vi "CallVI.vi"(1 "Output Names":string[](array[string]), 2 "Input Values":variant[](array[variant]), 3 "Input Names":string[](array[string]), 4 "VI":refnum<vi>) -> (0 "Output Values":variant[](array[variant]))   [LabVIEW 2014]
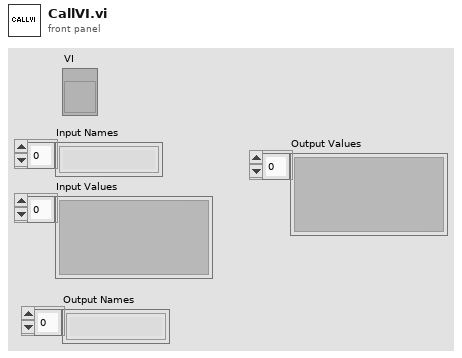
[diagram p1: front panel]
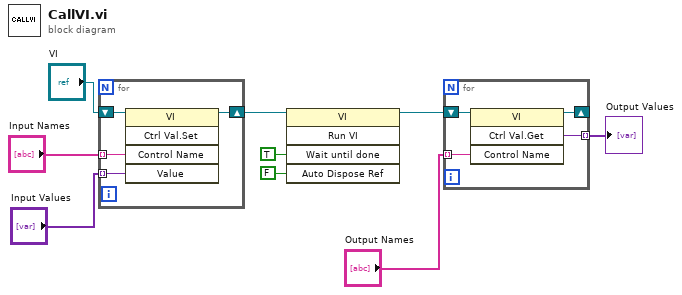
[diagram p0: block diagram]
diagram:
  n1 = for {
    tunnel: "Input Names" -> [w13] mode=indexing
    tunnel: "Input Values" -> [w12] mode=indexing
    shift-right: [w11] -> w9
    shift-left: "VI" -> [w10]
    n2 = invoke class="VI" method="Ctrl Val.Set"(reference=w10, "Control Name"=w13, "Value"=w12) -> (reference out=w11:refnum<vi>)  [unwired: 2 in, 4 out]
  }
  n3 = invoke class="VI" method="Run VI"(reference=w9, "Wait until done"=TRUE ("Wait Until Done"), "Auto Dispose Ref"=FALSE ("Auto Dispose Reference")) -> (reference out=w3:refnum<vi>)  [unwired: 2 in, 4 out]
  n4 = for {
    tunnel: "Output Names" -> [w16] mode=indexing
    tunnel: [w15] -> w1 mode=indexing
    shift-right: [w14] -> _
    shift-left: w3 -> [w17]
    n5 = invoke class="VI" method="Ctrl Val.Get"(reference=w17, "Control Name"=w16) -> (reference out=w14:refnum<vi>, "Get Control Value Variant"=w15:variant)  [unwired: 2 in, 2 out]
  }
  "Output Values" <- w1
